vi "TestInitialOutput.vi"(10 "Delay Time (s)":dbl=0.4) -> (0 "Current output (mA)":dbl, 1 "Current (mA) level\nfor output pins":dbl[](array[numeric]), 2 "Delay Time":dbl)   [LabVIEW 2018]
uses:
  GlobalVariables/WaveformCharGlobal.vi
  <vilib>/express/express arith-compare/Formula/XNode/ExpressFormulaBlockNode.xnode
panel:
  in  "Fixed Resistor":dbl=350.0
  out "MUX channel":i32
  in  "stop":bool
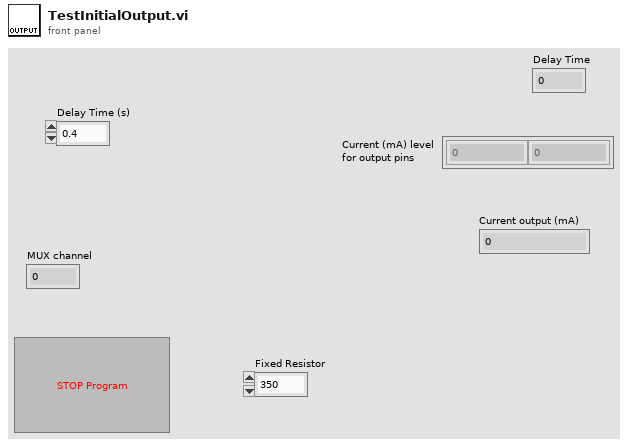
[diagram p1: front panel]
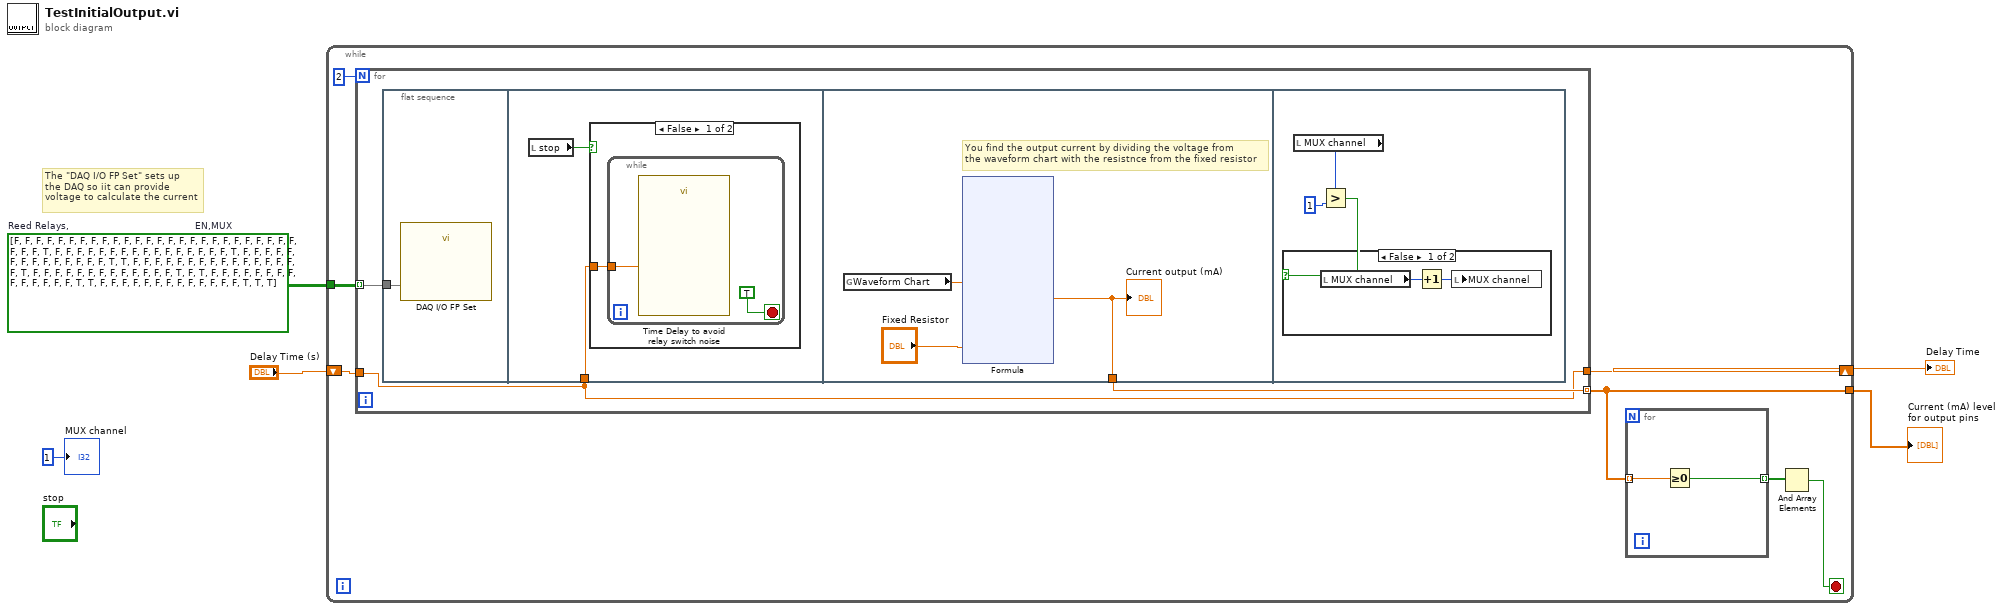
[diagram p0: block diagram]
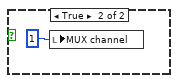
[diagram p3: hidden frame]
diagram:
  w4 = bool[][] [[FALSE, FALSE, FALSE, FALSE, FALSE, FALSE, FALSE, FALSE, FALSE, FALSE, FALSE, FALSE, FALSE, FALSE, FALSE, FALSE], [FALSE, FALSE, FALSE, FALSE, FALSE, FALSE, FALSE, FALSE, FALSE, FALSE, FALSE, FALSE, FALSE, TRUE, FALSE, FALSE], [FALSE, FALSE, FALSE, FALSE, FALSE, FALSE, FALSE, FALSE, FALSE, FALSE, FALSE, FALSE, FALSE, FALSE, TRUE, FALSE], [FALSE, FALSE, FALSE, FALSE, FALSE, FALSE, FALSE, FALSE, FALSE, FALSE, FALSE, FALSE, FALSE, TRUE, TRUE, FALSE], [FALSE, FALSE, FALSE, FALSE, FALSE, FALSE, FALSE, FALSE, FALSE, FALSE, FALSE, FALSE, FALSE, FALSE, FALSE, TRUE], [FALSE, FALSE, FALSE, FALSE, FALSE, FALSE, FALSE, FALSE, FALSE, FALSE, FALSE, FALSE, FALSE, TRUE, FALSE, TRUE], [FALSE, FALSE, FALSE, FALSE, FALSE, FALSE, FALSE, FALSE, FALSE, FALSE, FALSE, FALSE, FALSE, FALSE, TRUE, TRUE], [FALSE, FALSE, FALSE, FALSE, FALSE, FALSE, FALSE, FALSE, FALSE, FALSE, FALSE, FALSE, FALSE, TRUE, TRUE, TRUE]]  # Reed Relays,                                          EN,MUX
  # "The \"DAQ I/O FP Set\" sets up \nthe DAQ so iit can provide \nvoltage to calculate the current"
  n1 = while {
    tunnel: [w8] -> w5
    tunnel: w4 -> [w12]
    shift-right: [w9] -> w1
    shift-left: "Delay Time (s)" -> [w10]
    stop <- w6 stop-if-true
    n2 = for {
      N: 2 -> [_]
      tunnel: w12 -> [w17] mode=indexing
      tunnel: [w16] -> w8 mode=indexing
      tunnel: w10 -> [w15]
      tunnel: [w15] -> w9
      n3 = flat-sequence {
        tunnel: w17 -> [w18]
        tunnel: w15 -> [w19]
        tunnel: [w24] -> w16
        frame #0 {
          n4 = call "DAQ I/O FP Set"("data"=w18) -> ()  [unwired: 17 in, 2 out]
        }
        frame #1 {
          n5 = local read "stop"() -> (w20:bool)
          n6 = case shown="False" w20 {
            tunnel: w19 -> [w21 _]
            frame False {
              n7 = while {
                tunnel: w21 -> [w22]
                stop <- TRUE stop-if-true
                n8 = call "Time Delay to avoid relay switch noise"("Delay Time (s)"=w22) -> ()  [unwired: 10 in, 1 out]
              }
            }
            frame True {
            }
          }
        }
        frame #2 {
          # "You find the output current by dividing the voltage from \nthe waveform chart with the resistnce from the fixed resistor"
          n9 = global read "WaveformCharGlobal.vi" "Waveform Chart"() -> (w25:dbl)
          n10 = xnode "Formula"("X1"=w25, "X2"="Fixed Resistor") -> ("Result"=w24:dbl)  [unwired: 1 in, 1 out]
          "Current output (mA)" <- w24
        }
        frame #3 {
          n11 = local read "MUX channel"() -> (w38:i32)
          n12 = Greater?(x=w38, y=1) -> (0:w39:bool)
          n13 = case shown="False" w39 {
            frame False {
              n14 = local read "MUX channel"() -> (w41:i32)
              n15 = Increment(x=w41) -> (x+1=w40:i32)
              n16 = local write "MUX channel"(w40) -> ()
            }
            frame True {
              n17 = local write "MUX channel"(1 ("MUX channel")) -> ()
            }
          }
        }
      }
    }
    n18 = for {
      tunnel: w8 -> [w14] mode=indexing
      tunnel: [w13] -> w7 mode=indexing
      n19 = Greater Or Equal To 0?(x=w14) -> (x >= 0?=w13:bool)
    }
    n20 = And Array Elements(Boolean array=w7) -> (logical AND=w6:bool)
  }
  "Current (mA) level\nfor output pins" <- w5
  "Delay Time" <- w1
  "MUX channel" <- 1 ("MUX channel")
